vi "Fpga_v4.vi"() -> ()   [LabVIEW 2015]
uses:
  <vilib>/Platform/TimedLoop/XDataNode/timing_clust.ctl
  <vilib>/Platform/TimedLoop/XDataNode/nitl_modes.ctl
  <vilib>/Platform/TimedLoop/XDataNode/wakeup.ctl
  <vilib>/rvi/Emulation/niFpgaGetClockAttributes.vi
  <vilib>/rvi/Emulation/niFpgaSctlEmulationGetInTimedLoop.vi
  <vilib>/rvi/Emulation/niFpgaEmulationReportErrorSimple.vi
  <vilib>/rvi/eio/common/nirviEmuTemplateMethod_errors.vi
  <vilib>/rvi/Emulation/niFpgaCriticalErrorInLSC.vi
  <vilib>/rvi/interface/RandomDataEmulation/niFpgaRandomDataHandleErrors.vi
  <vilib>/eio/EIONode/EIONode.xnode
  <vilib>/Platform/TimedLoop/XDataNode/XDataNode.xnode
  <vilib>/rvi/DataTransferAndStorage/Container/XNode/niFpgaContainer.xnode
  <vilib>/rvi/interface/RandomDataEmulation/nirviRandomDataFpgaReadWriteTemplate.vi
  <vilib>/Platform/TimedLoop/XDataNode/XDNodeRunTimeDep.lvlib
panel:
  in  "Data write ON/OFF 2":bool
  in  "Data write ON/OFF":bool
  out "Mod2/DIO6_B":bool
  out "Timed Out?":bool
  out "x-y 3":u32
  in  "stop":bool
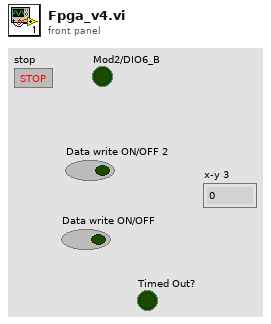
[diagram p1: front panel]
types:
  T1 = typedef "XDNodeRunTimeDep.lvlib/timing_clust.ctl" = cluster{"Expected End [f-1]":u64, "Actual End [f-1]":u64, "Finished Late? [f-1]":bool, "Expected End [i-1]":u64, "Actual End [i-1]":u64, "Finished Late? [i-1]":bool, "Expected Start [i]":u64, "Actual Start [i]":u64, "Expected Start [f]":u64, "Actual Start [f]":u64, "Source Name":string, "Structure Name":string, "Period":i64, "Deadline":i64, "Offset":i64, "Start":i64, "Priority":i32, "Timeout":i32, "Mode":T2, "Wakeup Reason":T3, "Error":errorcluster, "Source Type":string, "Secondary Source Type":string, "Global End Time":u64, "Global Start Time":u64, "Frame Duration":u64, "Iteration Duration":u64, "Assigned CPU":i32, "I/O Scan Engine Mode":u32}
  T2 = typedef "XDNodeRunTimeDep.lvlib/nitl_modes.ctl" = enum32{"No Change", "Process missed periods, maintain original phase", "Discard missed periods, maintain original phase", "Process missed periods, ignore original phase", "Discard missed periods, ignore original phase"}
  T3 = typedef "XDNodeRunTimeDep.lvlib/wakeup.ctl" = enum32{"Normal", "Aborted", "Asynchronous wakeup", "Timing source error", "Timed loop error", "Timeout"}
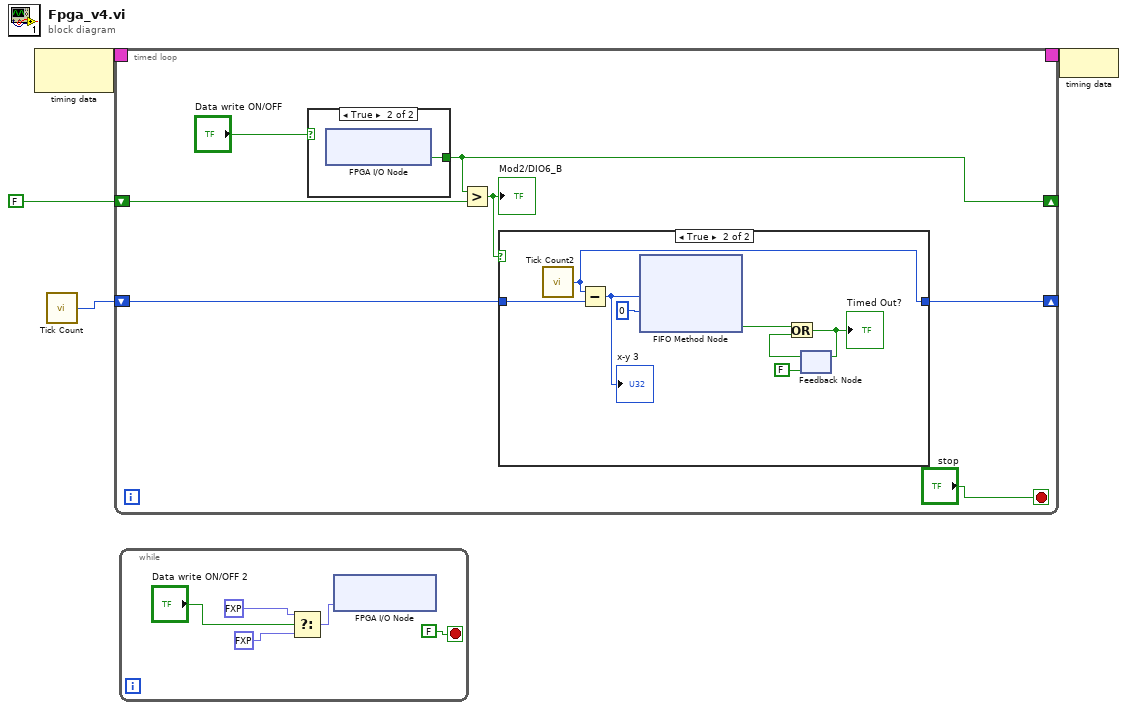
[diagram p0: block diagram]
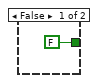
[diagram p3: hidden frame]
diagram:
  n1 = node-c288() -> (w4:T1)  [unwired: 1 in]
  n2 = call "Tick Count"() -> ("Tick Count(Ticks)"=w2:u32)
  n3 = timed-loop {
    shift-right: [w8] -> _
    shift-left: w2 -> [w9]
    shift-right: [w10] -> _
    shift-left: FALSE -> [w11]
    timing: w4 -> [_]
    timing-out: [_] -> w3
    stop <- "stop" stop-if-true
    n4 = case shown="True" "Data write ON/OFF" {
      tunnel: [FALSE ("Mod2/DIO6") w22] -> w10
      frame False {
      }
      frame True {
        n5 = xnode "FPGA I/O Node"() -> ("Mod2/DIO6"=w22:bool)  [unwired: 1 in, 1 out]
      }
    }
    n6 = Greater?(x=w10, y=w11) -> (0:w7:bool)
    "Mod2/DIO6_B" <- w7
    n7 = case shown="True" w7 {
      tunnel: w9 -> [w12 w15]
      tunnel: [w12 w14] -> w8
      frame False {
      }
      frame True {
        n8 = call "Tick Count2"() -> ("Tick Count(Ticks)"=w14:u32)
        n9 = Subtract(x=w14, y=w15) -> (x-y=w13:u32)
        "x-y 3" <- w13
        n10 = xnode ("FIFO Method Node")("Element"=w13, "Timeout"=0) -> ("Timed Out?"=w19:bool)  [unwired: 1 in, 1 out]
        n11 = feedback #1(FALSE) -> (w18:bool)
        n12 = Or(x=w19, y=w18) -> (x .or. y?=w16:bool)
        "Timed Out?" <- w16
        n13 = feedback-in #1(w16) -> ()
      }
    }
  }
  n14 = while {
    stop <- FALSE stop-if-true
    n15 = Select(t=fxp<+/-,20,5> 8.0 ("Mod4/AO0"), s="Data write ON/OFF 2", f=fxp<+/-,20,5> 0.0 ("Mod4/AO0")) -> (s? t:f=w25:fxp<+/-,20,5>)
    n16 = xnode "FPGA I/O Node"("Mod4/AO0"=w25) -> ()  [unwired: 1 in, 1 out]
  }
  n17 = node-c288(w3) -> ()
